vi "ADC_READ ADDOUT N-P.vi"(7 "Espera acceso FT":u32, 8 "Error IN":errorcluster, 10 "Sumador":u8, 11 "FTHandle IN":u32) -> (0 "Error OUT":errorcluster, 2 "ADDOUT":dbl, 3 "FTHandle OUT":u32)   [LabVIEW 2019]
uses:
  ASIC_Valores ADD_MUX_ena.ctl
  Global cuenta erroes.vi
  <vilib>/Analysis/NI_AALBase.lvlib
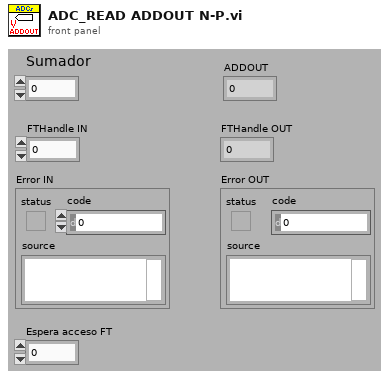
[diagram p1: front panel]
types:
  T1 = typedef "ASIC_Valores ADD_MUX_ena.ctl" = enum16{"---NULL--", "ADD A", "ADD B", "ADD C"}
  T2 = typedef "global erroes cluster.ctl" = cluster{"Errores FPGA":i32, "Errores Asic":i32, "Errores ADC adq":i32, "Errores ADC Asic":i32}
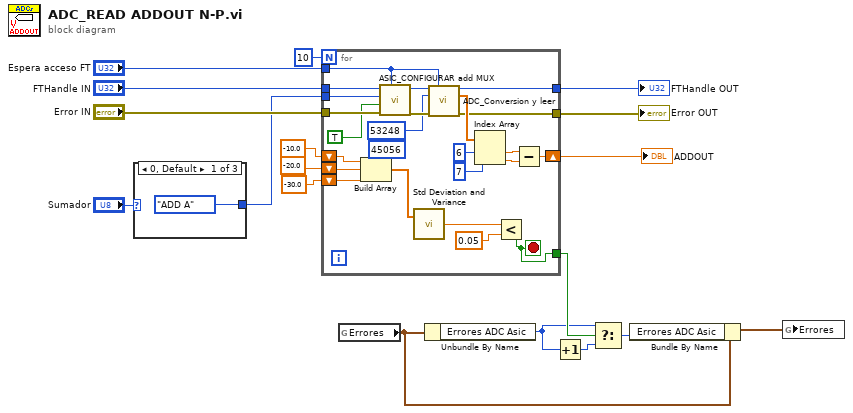
[diagram p0: block diagram]
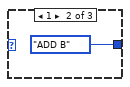
[diagram p2: hidden frame]
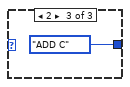
[diagram p3: hidden frame]
diagram:
  n1 = case shown="0, Default" "Sumador" {
    tunnel: [ASIC_Valores_ADD_MUX_ena."ADD A" ("ADD mux(0..3)") ASIC_Valores_ADD_MUX_ena."ADD B" ("ADD mux(0..3)") ASIC_Valores_ADD_MUX_ena."ADD C" ("ADD mux(0..3)")] -> w11
    frame 0, Default {
    }
    frame 1 {
    }
    frame 2 {
    }
  }
  n2 = for {
    N: 10 -> [_]
    tunnel: "Error IN" -> [w35]
    tunnel: "FTHandle IN" -> [w34]
    tunnel: "Espera acceso FT" -> [w33]
    tunnel: [w32] -> w13
    tunnel: [w31] -> w12
    tunnel: w11 -> [w29]
    shift-right: [w44] -> w18
    shift-left: -10.0 -> [w28]
    shift-left: -20.0 -> [w27]
    shift-left: -30.0 -> [w26]
    tunnel: [w22] -> w6
    stop <- w22 stop-if-true
    (unwired) u16 45056
    n3 = Build Array(w28, w27, w26) -> (w23:dbl[])
    n4 = call "ASIC_CONFIGURAR add MUX.vi"("Espera acceso USB"=w33, "error in"=w35, "BUFF_ENA"=TRUE, "ADD mux(0..3)"=w29, "ftHandle_in"=w34) -> ("error out"=w38:errorcluster, "ftHandle_out"=w37:u32)  [unwired: 5 in]
    n5 = call <vilib>:"Std Deviation and Variance.vi"("X"=w23) -> ("standard deviation"=w24:dbl)  [unwired: 1 in, 2 out]
    n6 = call "ADC_Conversion y leer.vi"("ftHandle_in 2"=w37, "Espera acceso USB"=w33, "Registro Conversion (0xD000)"=u16 53248, "error in 2"=w38) -> ("ftHandle_out"=w32:u32, "Datos Canal (V)"=w39:dbl[], "error out"=w31:errorcluster)  [unwired: 6 in, 3 out]
    n7 = Index Array(array=w39, index #1=6 ("index"), index #2=7 ("index")) -> (element #1=w42:dbl, element #2=w43:dbl)
    n8 = Less?(x=w24, y=0.05) -> (x < y?=w22:bool)
    n9 = Subtract(x=w42, y=w43) -> (x-y=w44:dbl)
  }
  "ADDOUT" <- w18
  "Error OUT" <- w12
  "FTHandle OUT" <- w13
  n10 = global read "Global cuenta erroes.vi" "Errores"() -> (w5:T2)
  n11 = Unbundle By Name(w5) -> ("Errores ADC Asic"=w3:i32)
  n12 = Increment(x=w3) -> (x+1=w2:i32)
  n13 = Select(t=w3, s=w6, f=w2) -> (s? t:f=w1:i32)
  n14 = Bundle By Name(cluster=w5, "Errores ADC Asic"=w1) -> (w4:T2)
  n15 = global write "Global cuenta erroes.vi" "Errores"(w4) -> ()
